vi "Test 2.vi"(8 "error in (no error)":errorcluster, 11 "Test Case In":refnum<class "Tests.lvclass">) -> (0 "error out":errorcluster, 3 "Test Case Out":refnum<class "Tests.lvclass">)   [LabVIEW 2021, in "Tests.lvclass"]
uses:
  Tests.lvclass
  C:/Program Files (x86)/National Instruments/LabVIEW 2021/vi.lib/Astemes/LUnit/Test Case.lvclass
  Proto/xmas.ctl
  <vilib>/Astemes/LUnit/Test Case.lvclass/Test Case.ctl
  4993e8ee-a06a-463a-9684-69129f64d5ce.vi
  <vilib>/Astemes/LUnit/Append Pass Result.vi
  <vilib>/Astemes/LUnit/Append Fail Result.vi
  <vilib>/Astemes/LUnit/Describe Comparison.vi
  <vilib>/Astemes/LUnit/Compare Variants.vi
  <vilib>/Astemes/LUnit/Variant to string.vi
  <vilib>/Utility/Data Type/Get Type Information.vi
  <vilib>/Utility/LVClass/Get LV Class Name.vi
  Tests.lvclass/Tests.ctl
  Proto/Rule.lvclass
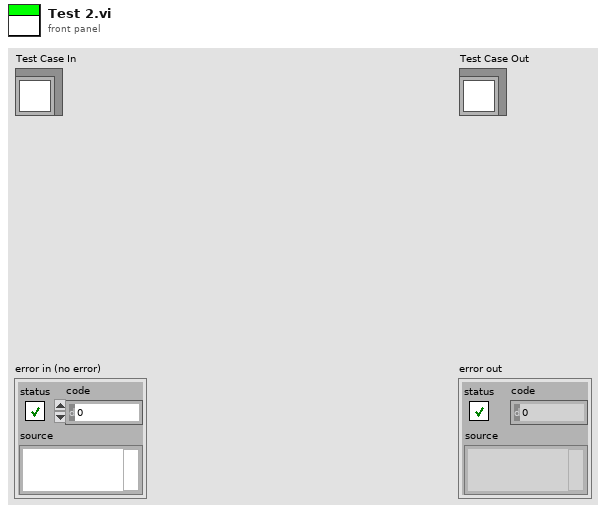
[diagram p1: front panel]
types:
  T1 = typedef "xmas.ctl" = cluster{"from":cluster{"x":u64, "m":u64, "a":u64, "s":u64}, "to":cluster{"x":u64, "m":u64, "a":u64, "s":u64}}
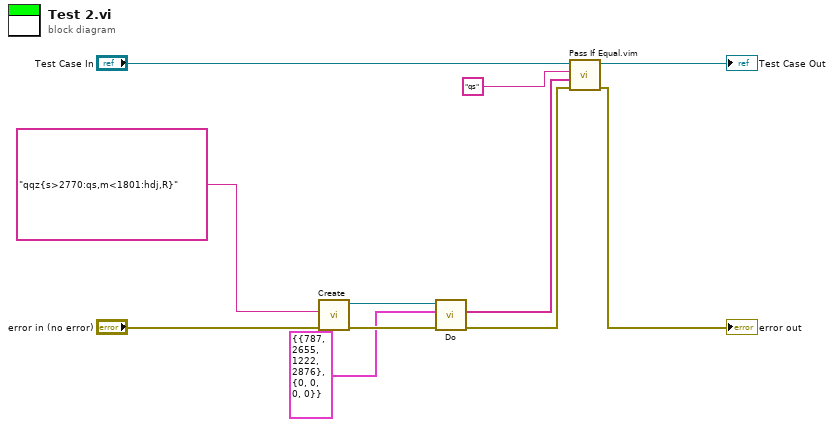
[diagram p0: block diagram]
diagram:
  n1 = call "Create.vi"("error in (no error)"="error in (no error)", "Input"="qqz{s>2770:qs,m<1801:hdj,R}") -> ("error out"=w7:errorcluster, "Proto"=w5:refnum<class "Rule.lvclass">)  [unwired: 7 in, 1 out]
  n2 = call "Do.vi"("error in (no error)"=w7, "In Range"=T1 {"from"={"x"=787, "m"=2655, "a"=1222, "s"=2876}, "to"={"x"=0, "m"=0, "a"=0, "s"=0}} ("Cluster"), "Rule In"=w5) -> ("error out"=w6:errorcluster, "Label"=w2:string[])  [unwired: 5 in, 2 out]
  n3 = call "Pass If Equal.vim"("error in (no error)"=w6, "Actual"=w2, "Expected"="qs" ("Label"), "LUnit Test Case In"="Test Case In") -> ("error out"=→"error out":errorcluster, "LUnit Test Case Out"=→"Test Case Out":refnum<class "Tests.lvclass">)  [unwired: 6 in]
